vi "Get Transfer Configuration.vi"(8 "error in (no error)":errorcluster, 11 "Component Configuration in":refnum<class "UDP Configurations.lvclass">=refnum) -> (0 "error out":errorcluster, 1 "Tx Transfer Configuration":refnum<class "Configuration.lvclass">, 2 "Rx Transfer Configuration":refnum<class "Configuration.lvclass">, 3 "Component Configuration out":refnum<class "UDP Configurations.lvclass">)   [LabVIEW 2020, in "UDP.lvlib" / "UDP Configurations.lvclass"]
uses:
  UDP Configurations.lvclass
  Rx Transfer/UDP Transfer Rx Configuration.lvclass
  Tx Transfer/UDP Transfer Tx Configuration.lvclass
  DSF Core.lvlibp/Classes/Configuration/Configuration.lvclass
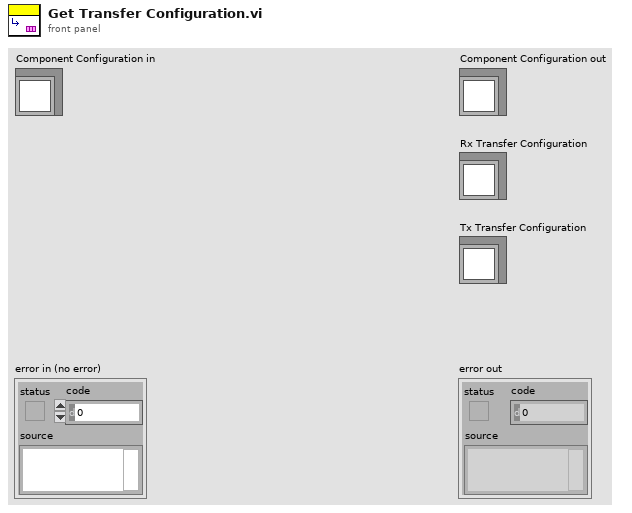
[diagram p1: front panel]
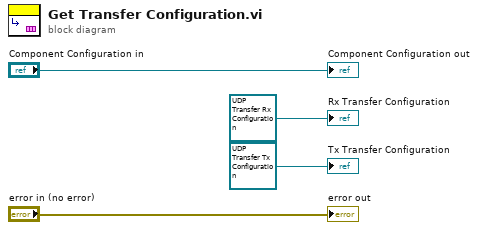
[diagram p0: block diagram]
diagram:
  "error out" <- "error in (no error)"
  "Component Configuration out" <- "Component Configuration in"
  "Rx Transfer Configuration" <- refnum<class "UDP Transfer Rx Configuration.lvclass"> refnum ("UDP Transceiver.lvlib:UDP Transfer Rx Configuration.lvclass")
  "Tx Transfer Configuration" <- refnum<class "UDP Transfer Tx Configuration.lvclass"> refnum ("UDP Transceiver.lvlib:UDP Transfer Tx Configuration.lvclass")
